vi "getKeyFormatFromTree.vi"(8 "error in":errorcluster, 10 "sec":string, 11 "Tree Refnum in":refnum<vi>) -> (0 "error out":errorcluster, 2 "keyFormat":string, 3 "Tree Refnum out":refnum<vi>)   [LabVIEW 2010]
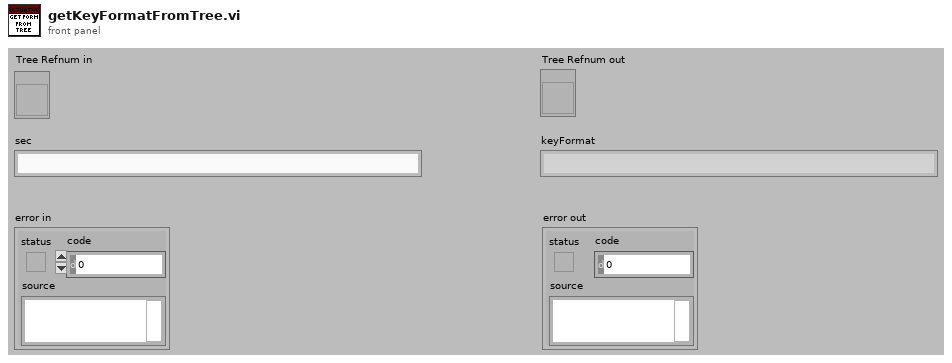
[diagram p1: front panel]
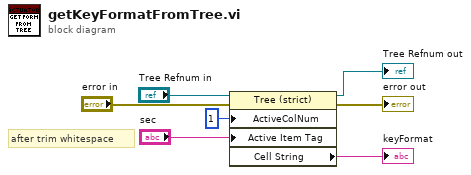
[diagram p0: block diagram]
diagram:
  # "after trim whitespace"
  n1 = property class="Tree (strict)"(reference="Tree Refnum in", error in="error in", "ActiveColNum"=1 ("Active Cell:Active Column Number"), "Active Item Tag"="sec") -> (reference out=→"Tree Refnum out":refnum<vi>, error out=→"error out":errorcluster, "Cell String"=→"keyFormat":string)
